vi "发送消息-重复数据.vi"(8 "错误输入（无错误）":errorcluster, 9 "数据":variant, 10 "消息组":string[](array[string]), 11 "输入队列":refnum<queue>) -> (0 "错误输出":errorcluster, 3 "输出队列":refnum<queue>)   [LabVIEW 2021, in "QueueLib.lvlib"]
uses:
  QueueLib.lvlib
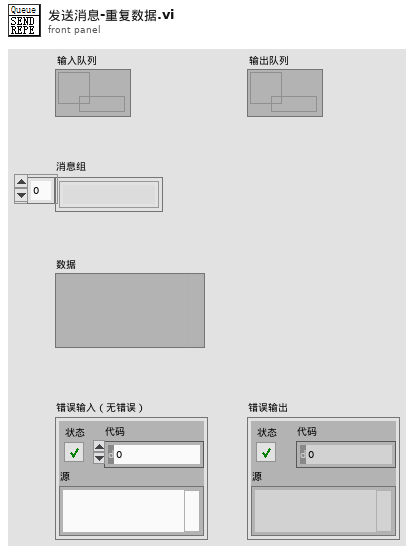
[diagram p1: front panel]
types:
  T1 = typedef "QueueLib.lvlib/数据类型.ctl" = cluster{"消息":string, "数据":variant}
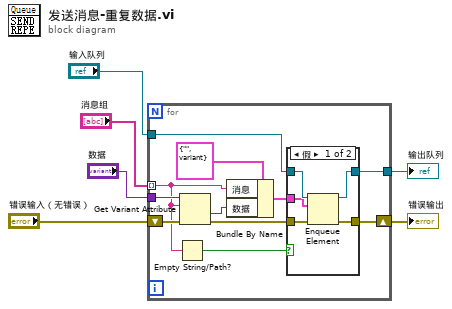
[diagram p0: block diagram]
diagram:
  n1 = for {
    tunnel: "数据" -> [w9]
    tunnel: "消息组" -> [w8] mode=indexing
    shift-right: [w14] -> w4
    shift-left: "错误输入（无错误）" -> [w15]
    tunnel: "输入队列" -> [w17]
    tunnel: [w13] -> w3
    n2 = Empty String/Path?(string/path=w8) -> (empty?=w11:bool)
    n3 = Get Variant Attribute(Variant=w9, name=w8, error in=w15) -> (value=w7:variant, error out=w10:errorcluster)  [unwired: 1 in, 2 out]
    n4 = Bundle By Name(cluster=T1 {"消息"="", "数据"=variant} ("数据类型"), "消息"=w8, "数据"=w7) -> (w16:T1)
    n5 = case shown="假" w11 {
      tunnel: w17 -> [w22 w23]
      tunnel: w16 -> [w21 _]
      tunnel: w10 -> [w20 w24]
      tunnel: [w19 w24] -> w14
      tunnel: [w18 w23] -> w13
      frame False {
        n6 = Enqueue Element(queue=w22, element=w21, error in (no error)=w20) -> (queue out=w18:refnum<queue>, error out=w19:errorcluster)  [unwired: 1 in, 1 out]
      }
      frame True {
      }
    }
  }
  "错误输出" <- w4
  "输出队列" <- w3
